vi "comparerecordandsave.vi"() -> ()   [LabVIEW 2020]
uses:
  common/record_file_handler/VFH-VNA_File_Handler.lvlib
  common/record_file_handler/VFH-file_cluster-NanoVNA.ctl
panel:
  in  "Checkbox":bool
  out "Raw":cluster{"Frequency":dbl[], "S21_Imag":dbl[]}[](graph)
  out "avg output 2":T1
  out "size(s) 2":i32
  in  "Folder Path 2":path=path "C:/NanoVNA-App/Recordings/2024-07-26 09-29-22"
  out "Data Points 2":i32
  out "avg output":T1
  out "size(s)":i32
  in  "Folder Path":path=path "C:/NanoVNA-App/Recordings/2024-07-26 09-29-22"
  out "Data Points":i32
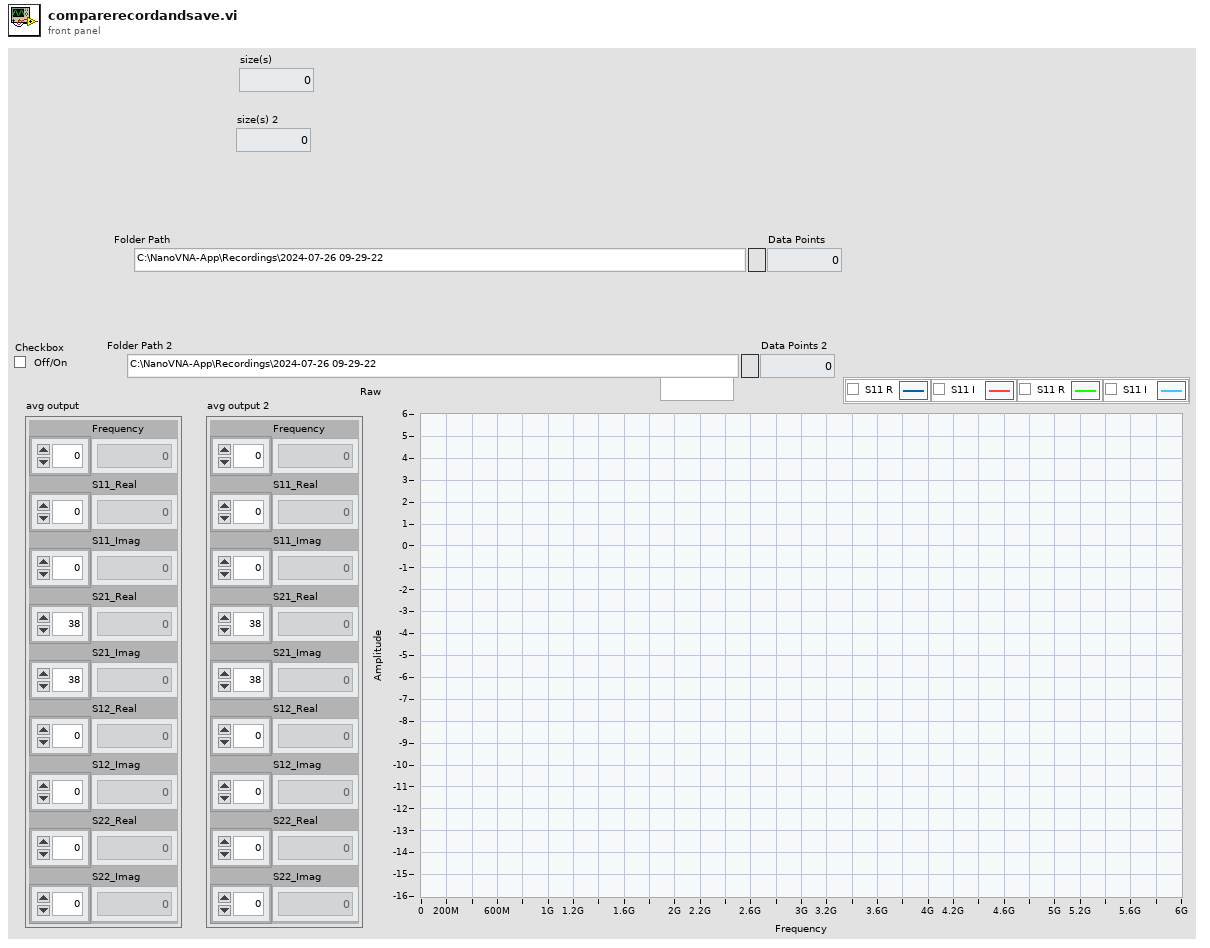
[diagram p1: front panel]
types:
  T1 = typedef "VFH-VNA_File_Handler.lvlib/VFH-file_cluster-NanoVNA.ctl" = cluster{"Frequency":dbl[], "S11_Real":dbl[], "S11_Imag":dbl[], "S21_Real":dbl[], "S21_Imag":dbl[], "S12_Real":dbl[], "S12_Imag":dbl[], "S22_Real":dbl[], "S22_Imag":dbl[]}
  T2 = typedef "VFH-VNA_File_Handler.lvlib/VFH-file_cluster-LabVIEWVNA.ctl" = cluster{"Frequency":dbl[], "S1_Real":dbl[], "S1_Imag":dbl[], "S11_Real":dbl[], "S11_Imag":dbl[], "S21_Real":dbl[], "S21_Imag":dbl[]}
  T3 = cluster{"S11'":cluster{"Frequency":dbl[], "S11_Real":dbl[]}, "S11''":cluster{"Frequency":dbl[], "S11_Real":dbl[]}, "Magnitude":cluster{"Frequency":dbl[], "Array":dbl[]}, "Eta":cluster{"Frequency":dbl[], "Array":dbl[]}, "Phase":cluster{"Frequency":dbl[], "Array":dbl[]}}
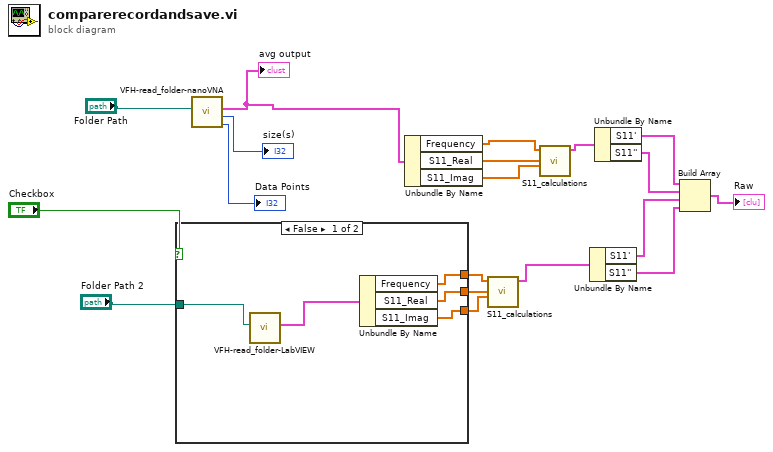
[diagram p0: block diagram]
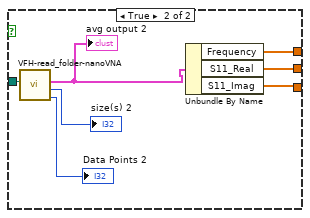
[diagram p2: hidden frame]
diagram:
  n1 = case shown="False" "Checkbox" {
    tunnel: "Folder Path 2" -> [w21 w31]
    tunnel: [w23 w28] -> w11
    tunnel: [w22 w27] -> w10
    tunnel: [w24 w25] -> w9
    frame False {
      n2 = call "VFH-read_folder-LabVIEW.vi"("Folder Path"=w21) -> ("avg output"=w20:T2)  [unwired: 8 in, 2 out]
      n3 = Unbundle By Name(w20) -> ("Frequency"=w24:dbl[], "S11_Real"=w23:dbl[], "S11_Imag"=w22:dbl[])
    }
    frame True {
      n4 = call "VFH-read_folder-nanoVNA.vi"("Folder Path"=w31) -> ("Data Points"=→"Data Points 2":i32, "size(s)"=→"size(s) 2":i32, "avg output"=w26:T1)  [unwired: 8 in]
      "avg output 2" <- w26
      n5 = Unbundle By Name(w26) -> ("Frequency"=w25:dbl[], "S11_Real"=w28:dbl[], "S11_Imag"=w27:dbl[])
    }
  }
  n6 = call "VFH-read_folder-nanoVNA.vi"("Folder Path"="Folder Path") -> ("Data Points"=→"Data Points":i32, "size(s)"=→"size(s)":i32, "avg output"=w12:T1)  [unwired: 8 in]
  "avg output" <- w12
  n7 = Unbundle By Name(w12) -> ("Frequency"=w15:dbl[], "S11_Real"=w13:dbl[], "S11_Imag"=w14:dbl[])
  n8 = call "S11_calculations.vi"("S11_Imag"=w10, "S11_Real"=w11, "Frequency"=w9) -> ("Raw"=w7:T3)  [unwired: 6 in, 2 out]
  n9 = call "S11_calculations.vi"("S11_Imag"=w14, "S11_Real"=w13, "Frequency"=w15) -> ("Raw"=w8:T3)  [unwired: 6 in, 2 out]
  n10 = Unbundle By Name(w7) -> ("S11'"=w4:cluster{"Frequency":dbl[], "S11_Real":dbl[]}, "S11''"=w3:cluster{"Frequency":dbl[], "S11_Real":dbl[]})
  n11 = Unbundle By Name(w8) -> ("S11'"=w6:cluster{"Frequency":dbl[], "S11_Real":dbl[]}, "S11''"=w5:cluster{"Frequency":dbl[], "S11_Real":dbl[]})
  n12 = Build Array(w6, w5, w4, w3) -> (→"Raw":cluster{"Frequency":dbl[], "S11_Real":dbl[]}[])
